vi "LOGfind.vi"(8 "Error In":errorcluster, 10 "Listener ID":string, 11 "Listeners In":refnum<queue>[](array[refnum])) -> (0 "Error Out":errorcluster, 2 "Index":i32, 3 "Listeners Out":refnum<queue>[](array[refnum]))   [LabVIEW 2025]
uses:
  LOGstatement.ctl
  <vilib>/Field R&D Services/Logger/Type Definitions/Tag.ctl
  <vilib>/Field R&D Services/Logger/Field_RnD_Services_Logger_Toolkit.lvlib
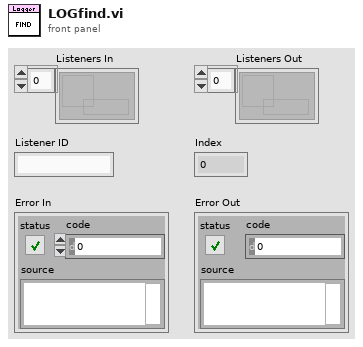
[diagram p1: front panel]
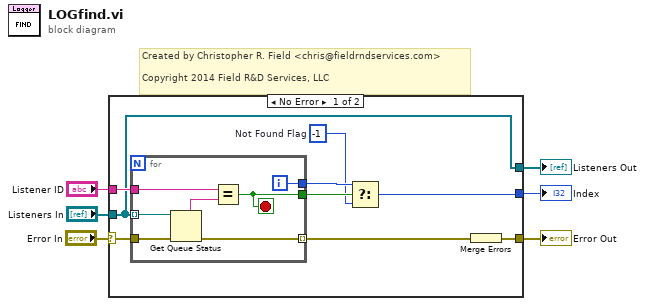
[diagram p0: block diagram]
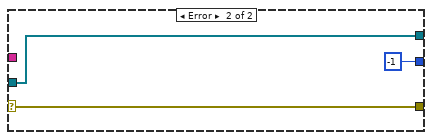
[diagram p2: hidden frame]
diagram:
  # "Created by Christopher R. Field <chris@fieldrndservices.com>\n\nCopyright 2014 Field R&D Services, LLC"
  n1 = case shown="No Error" "Error In" {
    selector: "Error In" -> [w8 w23]
    tunnel: "Listeners In" -> [w7 w25]
    tunnel: "Listener ID" -> [w15 _]
    tunnel: [w10 -1 ("Not Found Flag")] -> w4
    tunnel: [w9 w23] -> w3
    tunnel: [w7 w25] -> w1
    frame No Error {
      w11 = -1  # Not Found Flag
      n2 = for {
        tunnel: w7 -> [w22] mode=indexing
        tunnel: w8 -> [w21]
        tunnel: w15 -> [w20]
        tunnel: [w18] -> w14 mode=indexing
        tunnel: [w17] -> w13
        tunnel: [w16] -> w12
        i -> [w16]
        stop <- w17 stop-if-true
        n3 = Get Queue Status(queue=w22, error in (no error)=w21) -> (queue name=w19:string, error out=w18:errorcluster)  [unwired: 1 in, 6 out]
        n4 = Equal?(x=w20, y=w19) -> (x = y?=w17:bool)
      }
      n5 = Select(t=w12, s=w13, f=w11) -> (s? t:f=w10:i32)
      n6 = Merge Errors(w14) -> (w9:errorcluster)
    }
    frame Error {
    }
  }
  "Index" <- w4
  "Error Out" <- w3
  "Listeners Out" <- w1
